vi "VPA QC Assemble Checklist.vi"(10 "State Cluster":T1) -> (2 "State Cluster Out":T1)   [LabVIEW 2013]
uses:
  Controls/VPA QC State Data Cluster.ctl
  Controls/VPA QC General Cluster.ctl
  Controls/VPA QC State Enum.ctl
  Controls/VPA QC Bool Cluster.ctl
panel:
  in  "Done":bool
  in  "Voltage":bool caption="Ensure pump is running at the voltage specified by customer."
  in  "Wired":bool caption="Ensure that VPA is wired correctly."
  in  "Tighten Screws":bool
  in  "Drive Assem":bool caption="Ensure Drive Assembly checklist is complete."
  # "Drive Assembly Checklist"
  # "Assembly Checklist"
  # "Assembly Checklist"
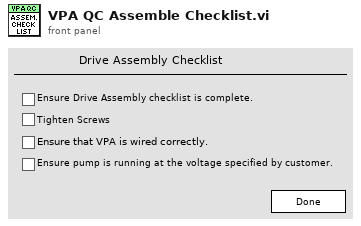
[diagram p1: front panel]
types:
  T1 = typedef "VPA QC State Data Cluster.ctl" = cluster{"XDCR 1":tag, "XDCR 2":tag, "General Information Clust":T2, "Assembly Checklist":cluster{"Ensure Drive Assembly checklist is completed.":bool, "Tighten Screws":bool, "Ensure VPA is wired correctly.":bool, "Ensure pump is running at voltage specified by customer.":bool}, "State":T3, "Manifold Leak Test Data":dbl[][], "Pressure Verification Test Data":dbl[][], "Flow Mode Verification Data":dbl[][], "DAQmx Error":errorcluster, "Bool Cluster":T4, "Leak Test Start Time":timestamp, "Pressure Test Start Time":timestamp, "Flow Test Start Time":timestamp, "Final Checklist cluster":cluster{"Check Fact Rest":bool, "Covers":bool, "Screws":bool, "Box":bool}, "Volts Constant":dbl, "Volume Constant A":dbl, "Volume Constant B":dbl, "Save File Path":path}
  T2 = typedef "VPA QC General Cluster.ctl" = cluster{"Tech Name":string, "Customer":string, "VPA Model":string, "G-72 Software Version":string, "Galil SN":string, "Galil Software Version":string, "VPA Serial Number":string, "Valve Serial Number":string, "A Side Transducer SN":string, "B Side Transducer SN":string, "A Side Motor SN":string, "B Side Motor SN":string, "A Side Gear Reducer SN":string, "B Side Gear Reducer SN":string, "A Side Limit Switch SN":string, "B Side Limit Switch Sn":string, "Pump Voltage":string, "Date":timestamp}
  T3 = typedef "VPA QC State Enum.ctl" = enum16{"General Information", "XDCR and LS Check", "Check Pump Function", "Manifold/Cylinder Leak Test", "Exit"}
  T4 = typedef "VPA QC Bool Cluster.ctl" = cluster{"Assembly":bool, "Gen":bool, "XDCR and LS Setup":bool, "Verify Pump Operation":bool, "Leak Test":bool, "Calibrate XDCRs":bool, "P Mode Verify":bool, "F Mode Verify":bool, "Vol Calibration":bool, "Final Checklist":bool}
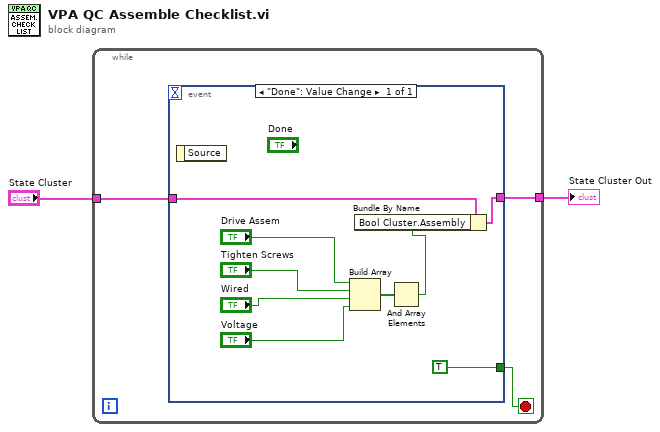
[diagram p0: block diagram]
diagram:
  n1 = while {
    tunnel: "State Cluster" -> [w4]
    tunnel: [w3] -> w1
    stop <- w5 stop-if-true
    n2 = event shown="[0] \"Done\": Value Change" {
      selector: _ -> [_]
      dyn-events: _ -> [_]
      timeout: _ -> [_]
      tunnel: [TRUE] -> w5
      tunnel: w4 -> [w8]
      tunnel: [w6] -> w3
      event "Done": Value Change {
        n3 = event-data() -> ()  [unwired: 1 in, 1 out]
        n4 = Build Array("Drive Assem", "Tighten Screws", "Wired", "Voltage") -> (w9:bool[])
        n5 = And Array Elements(Boolean array=w9) -> (logical AND=w7:bool)
        n6 = Bundle By Name(cluster=w8, "Bool Cluster.Assembly"=w7) -> (w6:T1)
      }
    }
  }
  "State Cluster Out" <- w1
